vi "Write Message Class Name.vi"(8 "Error In":errorcluster, 10 "Message Class Name":string, 11 "CS++LNAMessage in":refnum<class "CS++LNAMessage.lvclass">) -> (0 "Error Out":errorcluster, 3 "CS++LNAMessage out":refnum<class "CS++LNAMessage.lvclass">)   [LabVIEW 2014, in "CS++LNA.lvlib" / "CS++LNAMessage.lvclass"]
doc: "Write message class name to attribute."
uses:
  CS++LNAMessage.lvclass
  CS++LNAMessage.lvclass/CS++LNAMessage.ctl
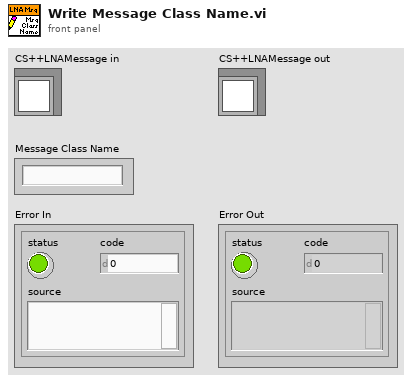
[diagram p1: front panel]
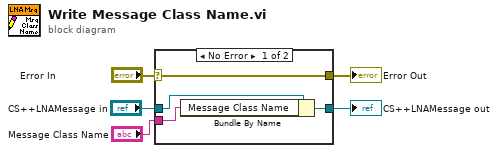
[diagram p0: block diagram]
diagram:
  n1 = case shown="No Error" "Error In" {
    selector: "Error In" -> [w9 w10]
    tunnel: [w9 w10] -> w4
    tunnel: [w7 w11] -> w2
    tunnel: "CS++LNAMessage in" -> [w8 w11]
    tunnel: "Message Class Name" -> [w6 _]
    frame No Error {
      n2 = Bundle By Name(cluster=w8, "Message Class Name"=w6) -> (w7:refnum<class "CS++LNAMessage.lvclass">)
    }
    frame Error {
    }
  }
  "Error Out" <- w4
  "CS++LNAMessage out" <- w2
